vi "MEMR-Process Frame.vi"(0 "State In":T1, 2 "queue data":cluster{bool, dbl[][], "Step Out":T2}, 7 "Analysis":T3, 11 "error in (no error)":errorcluster, 13 "controls":T4) -> (4 "State Out":T1, 8 "finished":bool, 15 "error out":errorcluster)   [LabVIEW 2020]
uses:
  Typedefs/MEMR-Controls.ctl
  Typedefs/MEMR-Analysis State.ctl
  Typedefs/MEMR-Analysis.ctl
  Typedefs/MEMR-Sequence Step.ctl
  <vilib>/Analysis/baseanly.llb/Mean.vi
  <vilib>/Analysis/baseanly.llb/Mean (DBL).vi
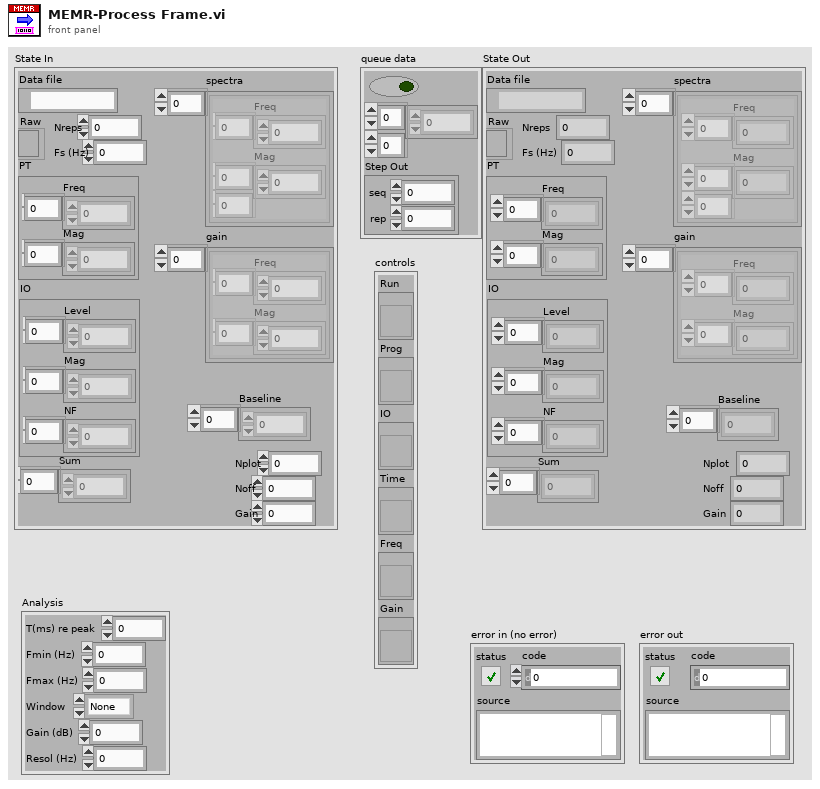
[diagram p1: front panel]
types:
  T1 = typedef "MEMR-Analysis State.ctl" = cluster{"Data file":path, "Raw":refnum<file>, "PT":cluster{"Freq":dbl[], "Mag":dbl[]}, "IO":cluster{"Level":dbl[], "Mag":dbl[], "NF":dbl[]}, "Nreps":i32, "Fs (Hz)":dbl, "Sum":dbl[], "Nplot":i32, "Noff":i32, "Gain":dbl, "spectra":cluster{"Freq":dbl[], "Mag":dbl[][]}[], "gain":cluster{"Freq":dbl[], "Mag":dbl[]}[], "Baseline":dbl[]}
  T2 = typedef "MEMR-Sequence Step.ctl" = cluster{"seq":i32, "rep":i32}
  T3 = typedef "MEMR-Analysis.ctl" = cluster{"T(ms) re peak":dbl, "Fmin (Hz)":dbl, "Fmax (Hz)":dbl, "Window":enum16{"None", "Hanning", "Hamming"}, "Gain (dB)":dbl, "Resol (Hz)":dbl}
  T4 = typedef "MEMR-Controls.ctl" = cluster{"Run":refnum<vi>, "Prog":refnum<vi>, "IO":refnum<vi>, "Time":refnum<vi>, "Freq":refnum<vi>, "Gain":refnum<vi>}
  T5 = enum16{"User", "Prism", "Kelly", "Dark2", "Sequential", "Hue"}
  T6 = cluster{"Freq (Hz)":dbl[], "+Freq. Mag of FFT (dB rms)":dbl[]}
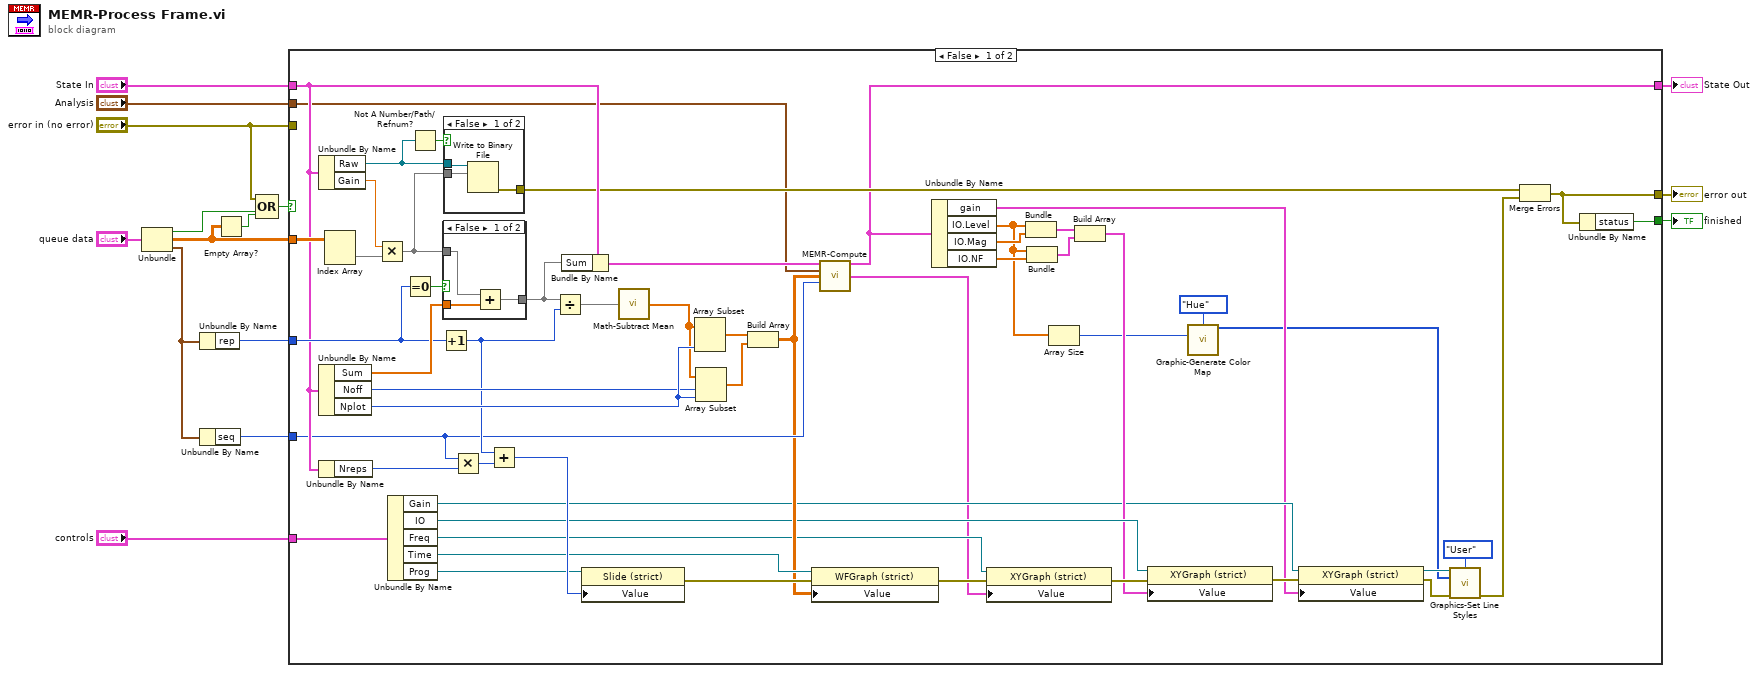
[diagram p0: block diagram]
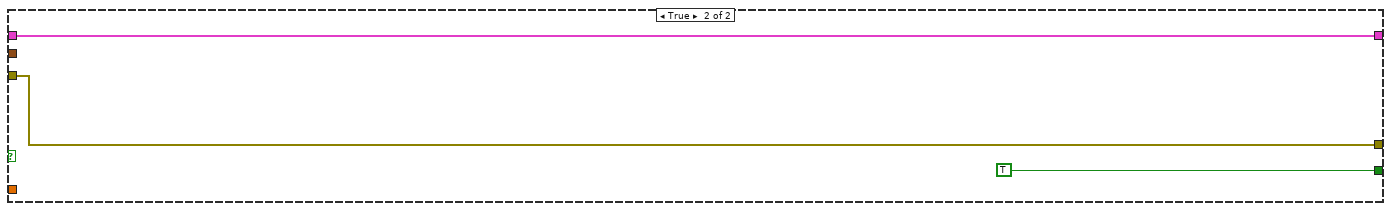
[diagram p4: hidden frame]
diagram:
  n1 = Unbundle("queue data") -> (w2:bool, w8:dbl[][], "Step Out"=w6:T2)
  n2 = Unbundle By Name(w6) -> ("rep"=w9:i32)
  n3 = Unbundle By Name(w6) -> ("seq"=w5:i32)
  n4 = Empty Array?(array=w8) -> (empty?=w3:bool)
  n5 = Compound Arithmetic op=OR("error in (no error)", w2, w3) -> (w7:bool)
  n6 = case shown="False" w7 {
    tunnel: "Analysis" -> [w46 _]
    tunnel: "State In" -> [w57 w79]
    tunnel: "controls" -> [w41 _]
    tunnel: [w44 w78] -> w14
    tunnel: [w48 TRUE] -> w15
    tunnel: "error in (no error)" -> [_ w78]
    tunnel: w8 -> [w69 _]
    tunnel: w9 -> [w58 _]
    tunnel: w5 -> [w45 _]
    tunnel: [w28 w79] -> w4
    frame False {
      n7 = Unbundle By Name(w57) -> ("Raw"=w65:refnum<file>, "Gain"=w35:dbl)
      n8 = Unbundle By Name(w57) -> ("Sum"=w67:dbl[], "Noff"=w61:i32, "Nplot"=w62:i32)
      n9 = Unbundle By Name(w57) -> ("Nreps"=w56:i32)
      n10 = Index Array(array=w69) -> (element=w64:dbl[])  [unwired: 2 in]
      n11 = Multiply(x=w35, y=w64) -> (x*y=w36:dbl[])
      n12 = Unbundle By Name(w41) -> ("Gain"=w27:refnum<vi>, "IO"=w37:refnum<vi>, "Freq"=w39:refnum<vi>, "Time"=w51:refnum<vi>, "Prog"=w52:refnum<vi>)
      n13 = Equal To 0?(x=w58) -> (x = 0?=w68:bool)
      n14 = Not A Number/Path/Refnum?(number/path/refnum=w65) -> (NaN/Path/Refnum?=w66:bool)
      n15 = Increment(x=w58) -> (x+1=w54:i32)
      n16 = case shown="False" w68 {
        tunnel: w36 -> [w75 w76]
        tunnel: w67 -> [w74 _]
        tunnel: [w73 w76] -> w63
        frame False {
          n17 = Add(x=w75, y=w74) -> (x+y=w73:dbl[])
        }
        frame True {
        }
      }
      n18 = case shown="False" w66 {
        tunnel: w65 -> [w72 _]
        tunnel: w36 -> [w71 _]
        tunnel: [w70 _] -> w49
        frame False {
          n19 = Write to Binary File(file (use dialog)=w72, data=w71) -> (error out=w70:errorcluster)  [unwired: 4 in, 2 out]
        }
        frame True {
        }
      }
      n20 = Multiply(x=w45, y=w56) -> (x*y=w55:i32)
      n21 = Add(x=w54, y=w55) -> (x+y=w53:i32)
      n22 = Divide(x=w63, y=w54) -> (x/y=w42:dbl[])
      n23 = Bundle By Name(cluster=w57, "Sum"=w63) -> (w47:T1)
      n24 = property class="Slide (strict)"(reference=w52, "Value"=w53) -> (error out=w50:errorcluster)  [unwired: 1 in, 1 out]
      n25 = call "Math-Subtract Mean.vi"("Y"=w42) -> ("Y - mean(Y)"=w34:dbl[])  [unwired: 4 in]
      n26 = Array Subset(array=w34, length=w62) -> (w60:dbl[])  [unwired: 1 in]
      n27 = Array Subset(array=w34, index=w61, length=w62) -> (w59:dbl[])
      n28 = Build Array(w60, w59) -> (w43:dbl[][])
      n29 = property class="WFGraph (strict)"(reference=w51, error in=w50, "Value"=w43) -> (error out=w40:errorcluster)  [unwired: 1 out]
      n30 = call "MEMR-Compute.vi"("State In"=w47, "Analysis"=w46, "Avg"=w43, "seqIndex"=w45) -> ("State Out"=w28:T1, "freq response"=w25:T6)  [unwired: 10 in]
      n31 = Unbundle By Name(w28) -> ("gain"=w24:cluster{"Freq":dbl[], "Mag":dbl[]}[], "IO.Level"=w19:dbl[], "IO.Mag"=w32:dbl[], "IO.NF"=w33:dbl[])
      n32 = property class="XYGraph (strict)"(reference=w39, error in=w40, "Value"=w25) -> (error out=w38:errorcluster)  [unwired: 1 out]
      n33 = Bundle("Level"=w19, "Mag"=w32) -> (w31:cluster{"Level":dbl[], "Mag":dbl[]})  [unwired: 1 in]
      n34 = Bundle("Level"=w19, "NF"=w33) -> (w30:cluster{"Level":dbl[], "NF":dbl[]})  [unwired: 1 in]
      n35 = Array Size(array=w19) -> (size(s)=w17:i32)
      n36 = Build Array(w31, w30) -> (w29:cluster{"Level":dbl[], "NF":dbl[]}[])
      n37 = property class="XYGraph (strict)"(reference=w37, error in=w38, "Value"=w29) -> (error out=w26:errorcluster)  [unwired: 1 out]
      n38 = call "Graphic-Generate Color Map.vi"("Map"=T5."Hue", "Size"=w17) -> ("Colors"=w16:u32[])  [unwired: 13 in]
      n39 = property class="XYGraph (strict)"(reference=w27, error in=w26, "Value"=w24) -> (reference out=w23:refnum<vi>, error out=w22:errorcluster)
      n40 = call "Graphics-Set Line Styles.vi"("XY Graph"=w23, "Map"=T5."User", "Colors"=w16, "error in (no error)"=w22) -> ("error out"=w21:errorcluster)  [unwired: 10 in, 1 out]
      n41 = Merge Errors(w49, w21) -> (w44:errorcluster)
      n42 = Unbundle By Name(w44) -> ("status"=w48:bool)
    }
    frame True {
    }
  }
  "finished" <- w15
  "error out" <- w14
  "State Out" <- w4
